vi "Converter.vi"() -> ()   [LabVIEW 2022 SP3]
uses:
  #typedef_PXD_FileWritingOption.ctl
panel:
  in  "Export (use dialog)":path=path "C:/Users/User/Desktop/measurements/lnpix/2022-11-08_porownanie_szumow_zasilacze_kontrolery/4_PXI/ENC_LNPIX_dla_MZ/KRUM_0_gateTime_5s_onlyLow16bit_litle_endian.bin"
  in  "WritingOptions":T1=enum."OnlyLow16bit"
  in  "Immport":path=path "C:/Users/User/Desktop/measurements/lnpix/2022-11-08_porownanie_szumow_zasilacze_kontrolery/4_PXI/ENC_LNPIX_dla_MZ/KRUM_0_gateTime_5s_onlyLow16bit_litle_endian.bin"
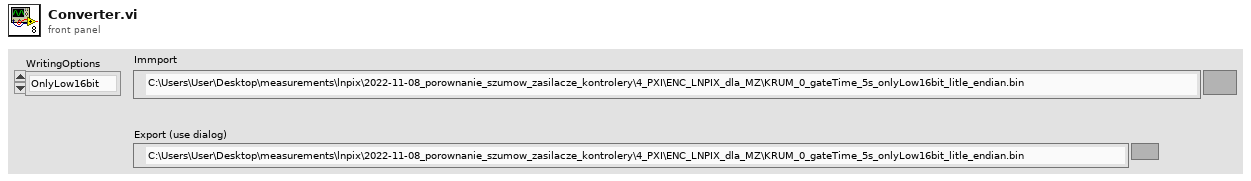
[diagram p1: front panel]
types:
  T1 = typedef "#typedef_PXD_FileWritingOption.ctl" = enum16{"OnlyLow32bit", "OnlyLow16bit", "OnlyHigh16bit", "High&Low16bit", "High&Low32bit"}
  T2 = enum16{"big-endian, network order", "native, host order", "little-endian"}
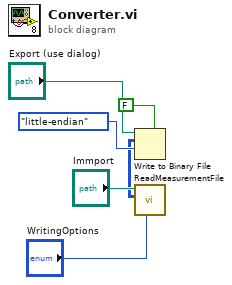
[diagram p0: block diagram]
diagram:
  n1 = call "ReadMeasurementFile.vi"("WritingOptions"="WritingOptions", "Path"="Immport") -> ("ThrScan_RICE_Low"=w2:u16[][])  [unwired: 5 in, 4 out]
  n2 = Write to Binary File(file (use dialog)="Export (use dialog)", data=w2, 5:FALSE ("prepend array or string size? (T)"), 9:T2."little-endian" ("byte order (0:big-endian, network order)")) -> ()  [unwired: 2 in, 3 out]
